vi "get VTK num Y Coords.vi"(8 "error in (no error)":errorcluster) -> (0 "error out":errorcluster, 3 "function return":i32)   [LabVIEW 2019, in "libConvectionDiffusionWrapper.lvlib"]
doc: "int getVTK_numYCoords();"
uses:
  libConvectionDiffusionWrapper.lvlib
panel:
  # "*******************************************************************\nConvection Diffusion\n\nAuthor: Paul Zügel\nGCSC-Frankfurt am Main 2020\n\n*******************************************************************"
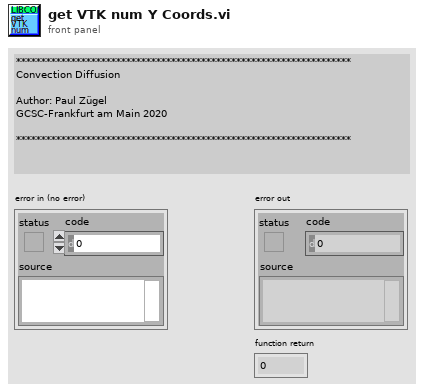
[diagram p1: front panel]
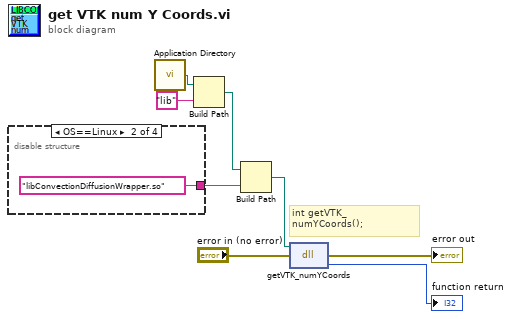
[diagram p0: block diagram]
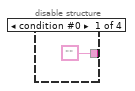
[diagram p2: hidden frame]
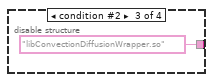
[diagram p3: hidden frame]
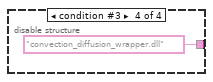
[diagram p4: hidden frame]
diagram:
  # "int getVTK_numYCoords();"
  n1 = disable-structure shown="OS==Linux" {
    disable-tunnel: ["" "libConvectionDiffusionWrapper.so" ("name or relative path") "libConvectionDiffusionWrapper.so" ("name or relative path") "convection_diffusion_wrapper.dll" ("name or relative path")] -> w2
    frame condition #0 {
    }
    frame condition #1 (active) {
    }
    frame condition #2 {
    }
    frame condition #3 {
    }
  }
  n2 = call <vilib>:"Application Directory.vi"() -> ("Application Directory"=w5:path)
  n3 = Build Path(base path=w5, name or relative path="lib") -> (appended path=w3:path)
  n4 = Build Path(base path=w3, name or relative path=w2) -> (appended path=w1:path)
  n5 = dll-call lib="home/paul/Schreibtisch/Convection_diffusion/LabView/lib/libConvectionDiffusionWrapper.*" fn="getVTK_numYCoords"(path in=w1, error in="error in (no error)") -> (error out=→"error out":errorcluster, "return type"=→"function return":i32)  [unwired: 1 in, 1 out]
